vi "VC840_Read.vi"(8 "error in (no error)":errorcluster, 11 "VISA resource name":refnum<visa-resource-name>) -> (0 "error out":errorcluster, 1 "Unit":string, 2 "Reading":dbl format="%.2f", 3 "VISA resource name out":refnum<visa-resource-name>, 4 "Status":T1, 5 "Mode":enum16{"?", "Diode", "Beep", "DC", "AC"}(ring))   [LabVIEW 2013]
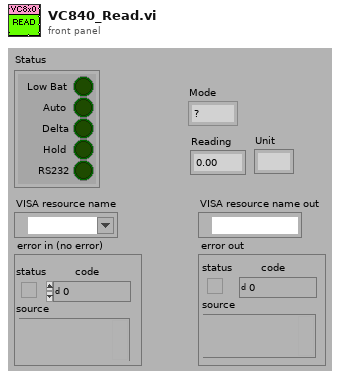
[diagram p1: front panel]
types:
  T1 = cluster{"Low Bat":bool, "Auto":bool, "Delta":bool, "Hold":bool, "RS232":bool}
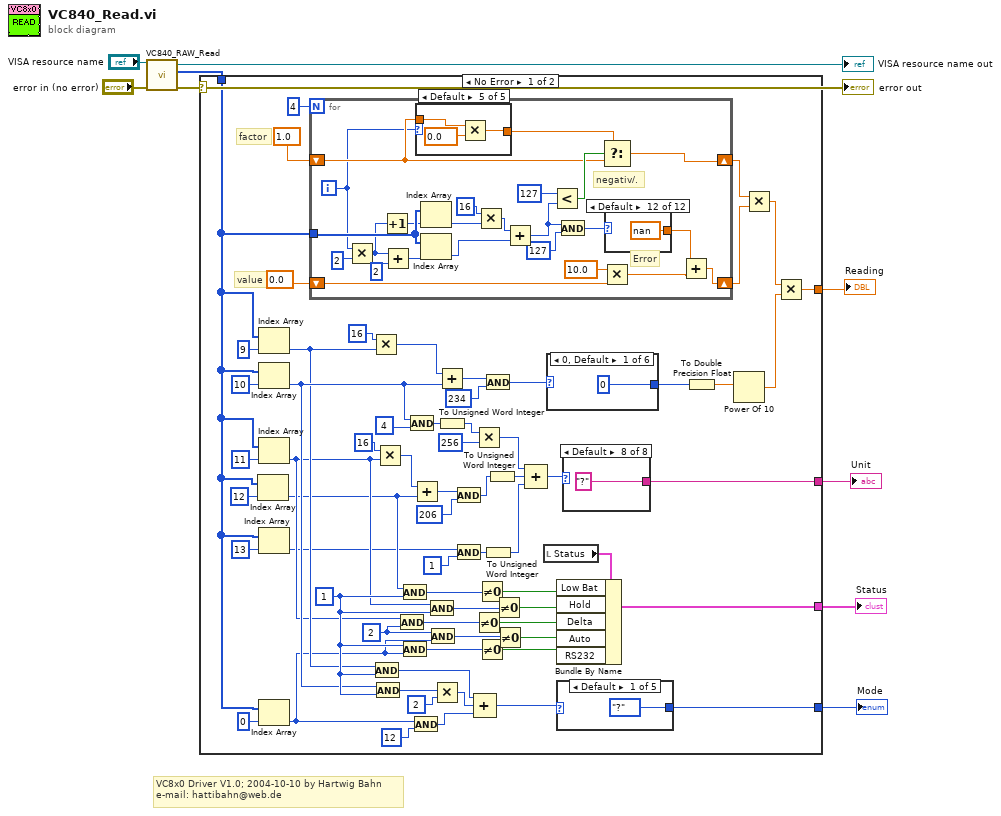
[diagram p0: block diagram]
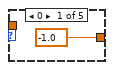
[diagram p2: hidden frame]
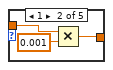
[diagram p3: hidden frame]
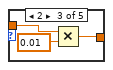
[diagram p4: hidden frame]
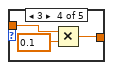
[diagram p5: hidden frame]
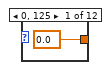
[diagram p6: hidden frame]
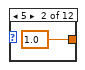
[diagram p7: hidden frame]
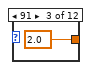
[diagram p8: hidden frame]
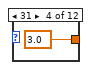
[diagram p9: hidden frame]
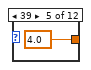
[diagram p10: hidden frame]
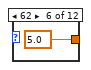
[diagram p11: hidden frame]
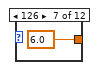
[diagram p12: hidden frame]
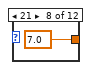
[diagram p13: hidden frame]
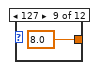
[diagram p14: hidden frame]
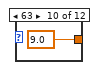
[diagram p15: hidden frame]
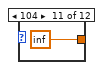
[diagram p16: hidden frame]
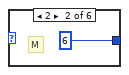
[diagram p17: hidden frame]
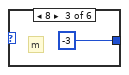
[diagram p18: hidden frame]
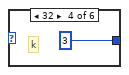
[diagram p19: hidden frame]
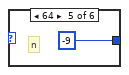
[diagram p20: hidden frame]
diagram:
  # "VC8x0 Driver V1.0; 2004-10-10 by Hartwig Bahn\ne-mail: hattibahn@web.de"
  n1 = call "VC840_RAW_Read.vi"("error in (no error)"="error in (no error)", "VISA resource name"="VISA resource name") -> ("error out"=w2:errorcluster, "Array"=w7:u8[], "VISA resource name out"=→"VISA resource name out":refnum<visa-resource-name>)  [unwired: 7 in]
  "error out" <- w2
  n2 = case shown="No Error" w2 {
    tunnel: [w75 enum16{"?", "Diode", "Beep", "DC", "AC"}."?"] -> w8
    tunnel: w7 -> [w52 _]
    tunnel: [w49 T1 {"Low Bat"=FALSE, "Auto"=FALSE, "Delta"=FALSE, "Hold"=FALSE, "RS232"=FALSE} ("Status")] -> w6
    tunnel: [w46 "?"] -> w1
    tunnel: [w27 nan] -> w3
    frame No Error {
      w69 = u8 1 ("y")
      w58 = u8 2 ("y")
      # "value"
      # "factor"
      n3 = Index Array(array=w52, index=12) -> (element=w61:u8)
      n4 = Index Array(array=w52, index=9) -> (element=w67:u8)
      n5 = Index Array(array=w52, index=10) -> (element=w68:u8)
      n6 = Index Array(array=w52, index=11) -> (element=w62:u8)
      n7 = Index Array(array=w52, index=13) -> (element=w40:u8)
      n8 = Index Array(array=w52, index=0) -> (element=w57:u8)
      n9 = for {
        N: 4 -> [_]
        tunnel: w52 -> [w93]
        shift-right: [w82] -> w19
        shift-left: 0.0 -> [w86]
        shift-right: [w80] -> w18
        shift-left: 1.0 -> [w78]
        i -> [w76]
        # "negativ/."
        n10 = Multiply(x=w76, y=2 ("x")) -> (x*y=w89:i32)
        n11 = Increment(x=w89) -> (x+1=w90:i32)
        n12 = Add(x=w89, y=2) -> (x+y=w87:i32)
        n13 = case shown="Default" w76 {
          tunnel: [-1.0 w101 w104 w107 w110] -> w79
          tunnel: w78 -> [_ w103 w106 w109 w112]
          frame 0 {
          }
          frame 1 {
            n14 = Multiply(x=w103, y=0.001) -> (x*y=w101:dbl)
          }
          frame 2 {
            n15 = Multiply(x=w106, y=0.01) -> (x*y=w104:dbl)
          }
          frame 3 {
            n16 = Multiply(x=w109, y=0.1) -> (x*y=w107:dbl)
          }
          frame Default {
            n17 = Multiply(x=w112, y=0.0) -> (x*y=w110:dbl)
          }
        }
        n18 = Index Array(array=w93, index=w90) -> (element=w92:u8)
        n19 = Index Array(array=w93, index=w87) -> (element=w91:u8)
        n20 = Multiply(x=u8 16, y=w92) -> (x*y=w96:u8)
        n21 = Add(x=w96, y=w91) -> (x+y=w94:u8)
        n22 = Less?(x=u8 127, y=w94) -> (x < y?=w81:bool)
        n23 = And(x=w94, y=u8 127) -> (x .and. y?=w95:u8)
        n24 = Select(t=w79, s=w81, f=w78) -> (s? t:f=w80:dbl)
        n25 = Multiply(x=10.0, y=w86) -> (x*y=w84:dbl)
        n26 = case shown="Default" w95 {
          tunnel: [0.0 1.0 2.0 3.0 4.0 5.0 6.0 7.0 8.0 9.0 inf sgl nan] -> w83
          frame 0, 125 {
          }
          frame 5 {
          }
          frame 91 {
          }
          frame 31 {
          }
          frame 39 {
          }
          frame 62 {
          }
          frame 126 {
          }
          frame 21 {
          }
          frame 127 {
          }
          frame 63 {
          }
          frame 104 {
          }
          frame Default {
            # "Error"
          }
        }
        n27 = Add(x=w83, y=w84) -> (x+y=w82:dbl)
      }
      n28 = Multiply(x=u8 16, y=w67) -> (x*y=w23:u8)
      n29 = And(x=w67, y=w69) -> (x .and. y?=w70:u8)
      n30 = And(x=w68, y=w69) -> (x .and. y?=w71:u8)
      n31 = Multiply(x=u8 16, y=w62) -> (x*y=w33:u8)
      n32 = And(x=w62, y=w58) -> (x .and. y?=w59:u8)
      n33 = And(x=w61, y=w69) -> (x .and. y?=w48:u8)
      n34 = And(x=w69, y=w57) -> (x .and. y?=w53:u8)
      n35 = And(x=w68, y=u8 4) -> (x .and. y?=w37:u8)
      n36 = And(x=w57, y=u8 12) -> (x .and. y?=w66:u8)
      n37 = Add(x=w33, y=w61) -> (x+y=w34:u8)
      n38 = And(x=w62, y=w69) -> (x .and. y?=w63:u8)
      n39 = And(x=w58, y=w57) -> (x .and. y?=w55:u8)
      n40 = Multiply(x=w71, y=u8 2) -> (x*y=w73:u8)
      n41 = Add(x=w23, y=w68) -> (x+y=w24:u8)
      n42 = To Unsigned Word Integer(number=w37) -> (unsigned 16bit integer=w12:u16)
      n43 = And(x=w34, y=u8 206) -> (x .and. y?=w43:u8)
      n44 = And(x=w40, y=u8 1) -> (x .and. y?=w42:u8)
      n45 = Multiply(x=w12, y=u16 256) -> (x*y=w44:u16)
      n46 = Not Equal To 0?(x=w59) -> (x != 0?=w60:bool)
      n47 = Compound Arithmetic op=ADD(w70, w73, w66) -> (w74:u8)
      n48 = Not Equal To 0?(x=w48) -> (x != 0?=w50:bool)
      n49 = Not Equal To 0?(x=w53) -> (x != 0?=w54:bool)
      n50 = And(x=w24, y=u8 234) -> (x .and. y?=w26:u8)
      n51 = To Unsigned Word Integer(number=w42) -> (unsigned 16bit integer=w11:u16)
      n52 = To Unsigned Word Integer(number=w43) -> (unsigned 16bit integer=w10:u16)
      n53 = Not Equal To 0?(x=w63) -> (x != 0?=w64:bool)
      n54 = Not Equal To 0?(x=w55) -> (x != 0?=w56:bool)
      n55 = Compound Arithmetic op=ADD(w44, w10, w11) -> (w45:u16)
      n56 = local read "Status"() -> (w14:T1)
      n57 = case shown="0, Default" w26 {
        tunnel: [0 6 -3 3 -9 -6] -> w47
        frame 0, Default {
        }
        frame 2 {
          # "M"
        }
        frame 8 {
          # "m"
        }
        frame 32 {
          # "k"
        }
        frame 64 {
          # "n"
        }
        frame 128 {
          # "µ"
        }
      }
      n58 = Bundle By Name(cluster=w14, "Low Bat"=w50, "Hold"=w64, "Delta"=w60, "Auto"=w56, "RS232"=w54) -> (w49:T1)
      n59 = case shown="Default" w74 {
        tunnel: [enum16{"?", "Diode", "Beep", "DC", "AC"}."?" enum16{"?", "Diode", "Beep", "DC", "AC"}."Diode" enum16{"?", "Diode", "Beep", "DC", "AC"}."Beep" enum16{"?", "Diode", "Beep", "DC", "AC"}."DC" enum16{"?", "Diode", "Beep", "DC", "AC"}."AC"] -> w75
        frame Default {
        }
        frame 1 {
        }
        frame 2 {
        }
        frame 4 {
        }
        frame 8 {
        }
      }
      n60 = case shown="Default" w45 {
        tunnel: ["°C" "Hz" "V" "A" "Ohm" "F" "%" "?"] -> w46
        frame 1 {
        }
        frame 2 {
        }
        frame 4 {
        }
        frame 8 {
        }
        frame 64 {
        }
        frame 128 {
        }
        frame 1024 {
        }
        frame Default {
        }
      }
      n61 = To Double Precision Float(number=w47) -> (double precision float=w13:dbl)
      n62 = Power Of 10(x=w13) -> (10^x=w28:dbl)
      n63 = Multiply(x=w18, y=w19) -> (x*y=w29:dbl)
      n64 = Multiply(x=w29, y=w28) -> (x*y=w27:dbl)
    }
    frame Error {
    }
  }
  "Mode" <- w8
  "Status" <- w6
  "Reading" <- w3
  "Unit" <- w1
